vi "Add Channel Prompt.vi"(7 "BLRL Type":T1, 10 "Available Channels":string[](array[string])) -> (1 "Cancelled":bool, 2 "Selected Channel":string)   [LabVIEW 2020, in "VolatusGUIElements.lvlib" / "BluelinesRedlines.lvclass"]
uses:
  BluelinesRedlines.lvclass
  VolatusGUI/BluelinesRedlines Source/BLRL Type.ctl
  0ec21dd6-ad01-423a-a77b-75ffb1806ba1.vi
  <vilib>/Comparison/Less/Less Functor/Less Functor.lvclass
  VolatusGUI/BluelinesRedlines Source/BluelinesRedlines Source.lvclass
panel:
  in  "Cancel":bool
  in  "Add":bool
  out "Prompt":string
  in  "Filter":string
  in  "List":i32(listbox)
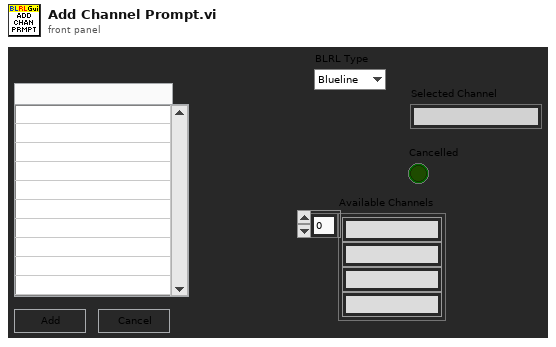
[diagram p1: front panel]
types:
  T1 = typedef "VolatusGUI.lvlib/BluelinesRedlines Source.lvclass/BLRL Type.ctl" = enum16{"Blueline", "Redline"}
  T2 = enum8{"Enabled", "Disabled", "Disabled and Grayed Out"}
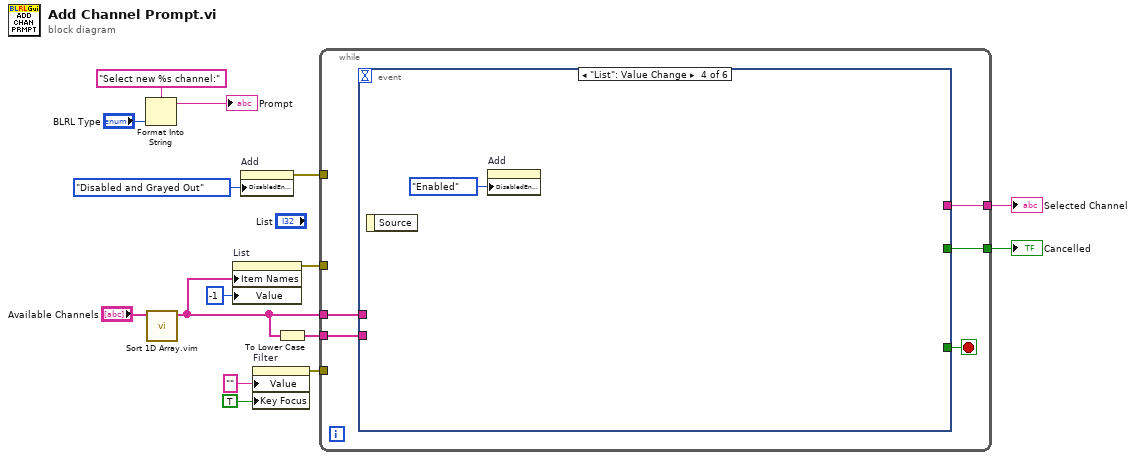
[diagram p0: block diagram]
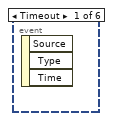
[diagram p2: hidden frame]
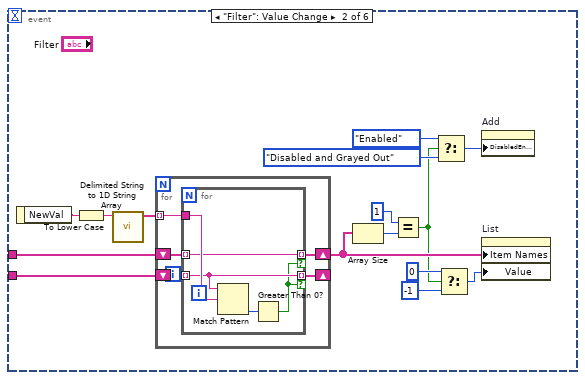
[diagram p3: hidden frame]
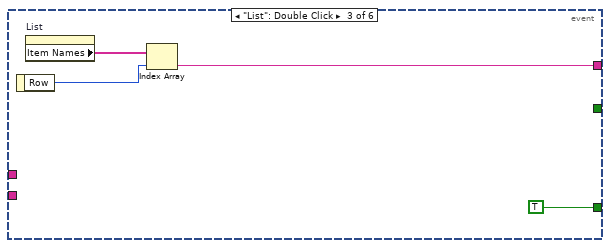
[diagram p4: hidden frame]
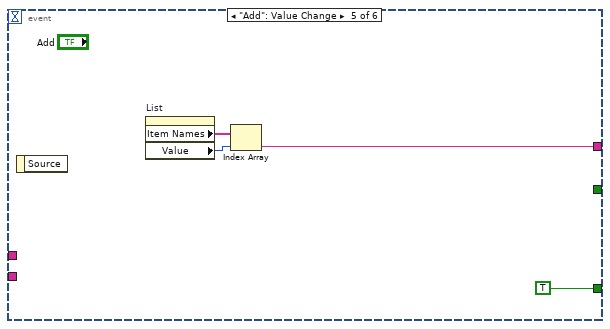
[diagram p5: hidden frame]
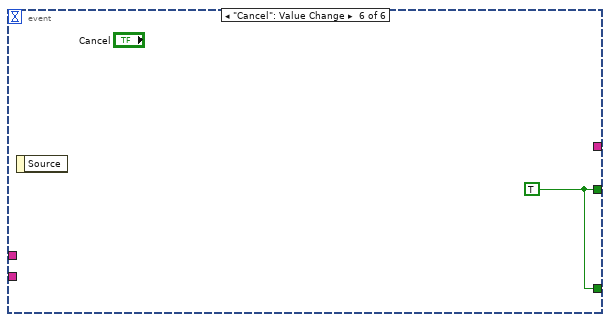
[diagram p6: hidden frame]
diagram:
  n1 = Format Into String(format string="Select new %s channel:" ("Prompt"), "BLRL Type") -> (resulting string=→"Prompt":string)  [unwired: 2 in, 1 out]
  n2 = call "Sort 1D Array.vim"("unsorted array"="Available Channels") -> ("sorted array"=w5:string[])  [unwired: 10 in]
  n3 = property on="List" class="LstBox (strict)"("Item Names"=w5, "Value"=-1 ("List")) -> (error out=w11:errorcluster)  [unwired: 2 in, 1 out]
  n4 = property on="Add" class="Bool"("DisabledEnum"=T2."Disabled and Grayed Out" ("Disabled")) -> (error out=w8:errorcluster)  [unwired: 2 in, 1 out]
  n5 = property on="Filter" class="Str"("Value"="" ("Filter"), "Key Focus"=TRUE) -> (error out=w2:errorcluster)  [unwired: 2 in, 1 out]
  n6 = To Lower Case(string=w5) -> (all lower case string=w4:string[])
  n7 = while {
    tunnel: w11 -> [_]
    tunnel: w5 -> [w20]
    tunnel: [w19] -> w10
    tunnel: w8 -> [_]
    tunnel: [w17] -> w6
    tunnel: w4 -> [w16]
    tunnel: w2 -> [_]
    stop <- w18 stop-if-true
    n8 = event shown="[3] \"List\": Value Change" {
      selector: _ -> [_ _ _ _ _ _]
      dyn-events: _ -> [_ _ _ _ _ _]
      timeout: _ -> [_ _ _ _ _ _]
      tunnel: w20 -> [_ w33 _ _ _ _]
      tunnel: [_ _ w47 _ w52 _] -> w19
      tunnel: [_ _ TRUE _ TRUE w55] -> w18
      tunnel: [_ _ _ _ _ w55] -> w17
      tunnel: w16 -> [_ w32 _ _ _ _]
      event Timeout {
        n9 = event-data() -> ()  [unwired: 1 in, 3 out]
      }
      event "Filter": Value Change {
        n10 = event-data() -> ("NewVal"=w35:string)  [unwired: 1 in]
        n11 = To Lower Case(string=w35) -> (all lower case string=w31:string)
        n12 = call <vilib>:"Delimited String to 1D String Array.vi"("delimited string"=w31) -> ("string array"=w34:string[])  [unwired: 10 in]
        n13 = for {
          tunnel: w34 -> [w38] mode=indexing
          shift-right: [w36] -> w30
          shift-left: w33 -> [w40]
          shift-right: [w37] -> _
          shift-left: w32 -> [w39]
          n14 = for {
            tunnel: w40 -> [w42] mode=indexing
            tunnel: w39 -> [w43] mode=indexing
            tunnel: w38 -> [w45]
            tunnel: [w43] -> w37 mode=indexing if=w41
            tunnel: [w42] -> w36 mode=indexing if=w41
            n15 = Match Pattern(string=w43, regular expression=w45) -> (offset past match=w44:i32)  [unwired: 1 in, 3 out]
            n16 = Greater Than 0?(x=w44) -> (x > 0?=w41:bool)
          }
        }
        n17 = Array Size(array=w30) -> (size(s)=w29:i32)
        n18 = Equal?(x=1, y=w29) -> (x = y?=w23:bool)
        n19 = Select(t=T2."Enabled", s=w23, f=T2."Disabled and Grayed Out" ("Disabled")) -> (s? t:f=w22:T2)
        n20 = Select(t=0, s=w23, f=-1) -> (s? t:f=w25:i32)
        n21 = property on="Add" class="Bool"("DisabledEnum"=w22) -> ()  [unwired: 2 in, 2 out]
        n22 = property on="List" class="LstBox (strict)"("Item Names"=w30, "Value"=w25) -> ()  [unwired: 2 in, 2 out]
      }
      event "List": Double Click {
        n23 = event-data() -> ("Row"=w48:i32)  [unwired: 1 in]
        n24 = property on="List" class="LstBox (strict)"() -> ("Item Names"=w49:string[])  [unwired: 2 in, 2 out]
        n25 = Index Array(array=w49, index=w48) -> (element=w47:string)
      }
      event "List": Value Change {
        n26 = event-data() -> ()  [unwired: 1 in, 1 out]
        n27 = property on="Add" class="Bool"("DisabledEnum"=T2."Enabled" ("Disabled")) -> ()  [unwired: 2 in, 2 out]
      }
      event "Add": Value Change {
        n28 = event-data() -> ()  [unwired: 1 in, 1 out]
        n29 = property on="List" class="LstBox (strict)"() -> ("Item Names"=w54:string[], "Value"=w53:i32)  [unwired: 2 in, 2 out]
        n30 = Index Array(array=w54, index=w53) -> (element=w52:string)
      }
      event "Cancel": Value Change {
        w55 = TRUE
        n31 = event-data() -> ()  [unwired: 1 in, 1 out]
      }
    }
  }
  "Selected Channel" <- w10
  "Cancelled" <- w6
